vi "Get Root Folder.vi"() -> (3 "Root folder":path)   [LabVIEW 2017, in "Front Panel Publisher.lvlib" / "Front Panel Manager.lvclass"]
uses:
  Front Panel Manager.lvclass
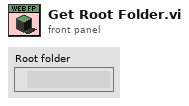
[diagram p1: front panel]
types:
  T1 = typedef "Front Panel Publisher.lvlib/Front Panel Manager.lvclass/Object Attributes.ctl" = cluster{"WebFrontPanels":refnum<class "Web Front Panel.lvclass">[], "WFP Names":string[], "Root folder":path, "Websocket Info":T2}
  T2 = typedef "Front Panel Publisher.lvlib/Front Panel Manager.lvclass/Websocket Info.ctl" = cluster{"Hostname":string, "Port":u16}
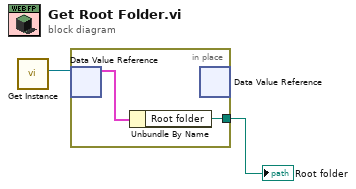
[diagram p0: block diagram]
diagram:
  n1 = call "Get Instance.vi"() -> ("DVRRefOut"=w1:refnum<data-value>)  [unwired: 7 in, 4 out]
  n2 = in-place {
    in-place-border: [w3] -> w2
    n3 = in-place-dvr #1(w1) -> (w4:T1)  [unwired: 1 out]
    n4 = Unbundle By Name(w4) -> ("Root folder"=w3:path)
    n5 = in-place-dvr #1() -> ()  [unwired: 1 in, 2 out]
  }
  "Root folder" <- w2
